vi "Get Logbook Entry.vi"(0 "VISA Session In":refnum<visa-resource-name>="OXYMAT", 1 "Target Address":u8=16 format="%.0x", 2 "Source Address":u8=208 format="%.0x", 7 "Entry":u8, 11 "error in (no error)":errorcluster) -> (4 "VISA Session Out":refnum<visa-resource-name>, 6 "Message Header":T2 {"Source Address" format="%.0x"; "Target Address" format="%.0x"}, 8 "Log Entry":T1 {"Timestamp" format="%<%X %x>T"}, 13 "Success":bool, 15 "error out":errorcluster)   [LabVIEW 2019, in "Siemens ELAN.lvlib"]
doc: "Using the Siemens ELAN protocol, gets the specifed log entry from the addressed analyzer. Also returns a boolean indicating that the addressed device provided a valid response.\n\n$Revision:: 0 $\n$Modtime:: yy-mm-dd hh:mm $\n$Author:: Dboyd $"
uses:
  Siemens ELAN.lvlib
  Message Header.ctl
  Channel Status.ctl
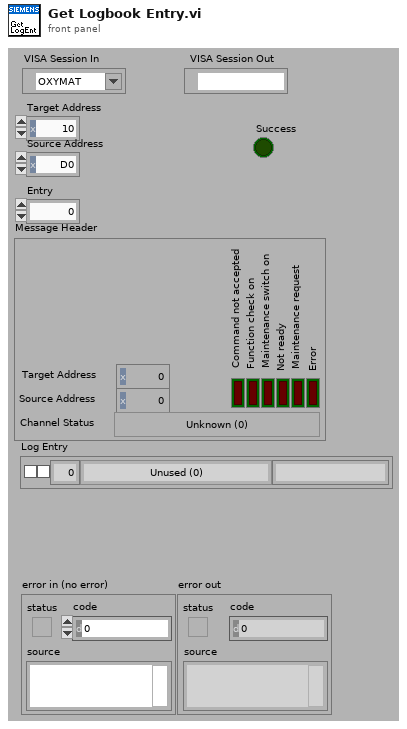
[diagram p1: front panel]
types:
  T1 = cluster{"Entry":u8, "Fault/Maint":enum8{"Unused (0)", "S1 Param Memory", "S2 Chopper/Magnetic Field", "S3 Microflow Sensor", "S4 External Fault", "S5 AnalyzerTemperature", "S6 Field Device Heater", "S7 Measuring Head Temperature", "S8 Pressure Sensor", "S9 Signal Too Large", "Unused (S10)", "S11 Reference Gas Supply", "S12 Mains Power", "Unused (S13)", "S14 Measured Value > Full Scale", "S15 Calibration Aborted", "S16 Sample Flow Too Low", "W1 Calibration Tolerance Violated", "W2 Zero Adjustment Too High", "W3 Slope/Sensitivity Too Small", "W4 Set Clock", "W5 Microflow Sensor", "W6 LCD Temperature", "W7 Analyzer/Receiver Temperature", "W8 Measuring Head Temperature", "W9 External Maintenance Request", "Unknown (W10)", "Unknown (W11)", "W12 Maintenance Check", "Unknown (>28)"}, "Appeared?":bool, "Acknowledged?":bool, "Timestamp":timestamp}
  T2 = typedef "Siemens ELAN.lvlib/Message Header.ctl" = cluster{"Target Address":u8, "Source Address":u8, "Error":bool, "Maintenance request":bool, "Not ready":bool, "Maintenance switch on":bool, "Function check on":bool, "Command not accepted":bool, "Channel Status":T3}
  T3 = typedef "Siemens ELAN.lvlib/Channel Status.ctl" = enum8{"Unknown (0)", "Warm-up", "Pause", "Standby", "Measure", "Zero calibration", "Adjust component slope", "Unknown (7)", "Adjust curve dip", "Adjust linearization sensitivity", "Adjust temperature compensation", "Adjust pressure compensation", "Adjust linearization zero", "Adjust flow sensor", "Autocal", "Adjust phase", "Zero calibration of O2 sensor", "Synchronous zero calibration", "Purging for synchronous zero calibration", "Adjust analog output", "Adjust analog input", "Cleaning", "Unknown (>21)"}
  T4 = enum8{"Unused (0)", "S1 Param Memory", "S2 Chopper/Magnetic Field", "S3 Microflow Sensor", "S4 External Fault", "S5 AnalyzerTemperature", "S6 Field Device Heater", "S7 Measuring Head Temperature", "S8 Pressure Sensor", "S9 Signal Too Large", "Unused (S10)", "S11 Reference Gas Supply", "S12 Mains Power", "Unused (S13)", "S14 Measured Value > Full Scale", "S15 Calibration Aborted", "S16 Sample Flow Too Low", "W1 Calibration Tolerance Violated", "W2 Zero Adjustment Too High", "W3 Slope/Sensitivity Too Small", "W4 Set Clock", "W5 Microflow Sensor", "W6 LCD Temperature", "W7 Analyzer/Receiver Temperature", "W8 Measuring Head Temperature", "W9 External Maintenance Request", "Unknown (W10)", "Unknown (W11)", "W12 Maintenance Check", "Unknown (>28)"}
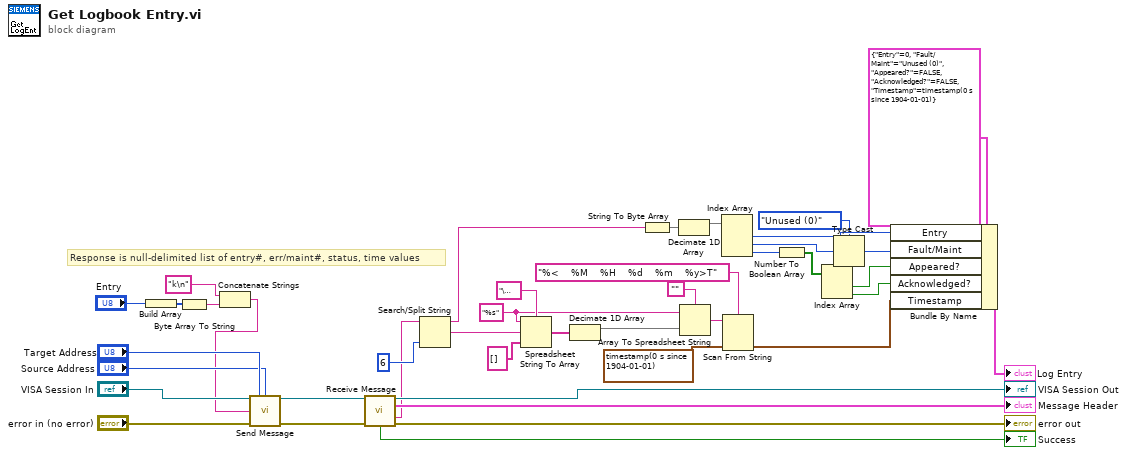
[diagram p0: block diagram]
diagram:
  w22 = "%s" ("format string")
  # "Response is null-delimited list of entry#, err/maint#, status, time values"
  n1 = Build Array("Entry") -> (w11:u8[])
  n2 = Byte Array To String(unsigned byte array=w11) -> (string=w10:string)
  n3 = Concatenate Strings("k\n" ("Command"), w10) -> (w8:string)
  n4 = call "Send Message.vi"("VISA Session In"="VISA Session In", "Target Address"="Target Address", "Source Address"="Source Address", "Command"=w8, "error in (no error)"="error in (no error)") -> ("VISA Session Out"=w41:refnum<visa-resource-name>, "error out"=w40:errorcluster)  [unwired: 8 in, 1 out]
  n5 = call "Receive Message.vi"("VISA Session In"=w41, "error in (no error)"=w40) -> ("VISA Session Out"=→"VISA Session Out":refnum<visa-resource-name>, "Message Header"=→"Message Header":T2, "Response"=w4:string, "Success"=→"Success":bool, "error out"=→"error out":errorcluster)  [unwired: 8 in, 1 out]
  n6 = Search/Split String(string=w4, offset (0)=6) -> (substring before match=w3:string, match + rest of string=w2:string)  [unwired: 1 in, 1 out]
  n7 = Spreadsheet String To Array(delimiter (Tab)="\u0000", format string=w22, spreadsheet string=w2, array type (2D Dbl)=string[] []) -> (array=w23:string[])
  n8 = Decimate 1D Array(w23) -> (w26:string[])  [unwired: 1 out]
  n9 = String To Byte Array(string=w3) -> (unsigned byte array=w7:u8[])
  n10 = Decimate 1D Array(w7) -> (w6:u8[])  [unwired: 1 out]
  n11 = Array To Spreadsheet String(delimiter (Tab)="", array=w26, 3:w22) -> (spreadsheet string=w28:string)
  n12 = Index Array(array=w6) -> (element #1=w20:u8, element #2=w24:u8, element #3=w18:u8)  [unwired: 3 in]
  n13 = Scan From String(format string="%<    %M    %H    %d    %m    %y>T", input string=w28, default 1=timestamp(0 s since 1904-01-01) ("Timestamp")) -> (output 1=w14:timestamp)  [unwired: 2 in, 3 out]
  n14 = Number To Boolean Array(number=w18) -> (Boolean array=w17:bool[])
  n15 = Index Array(array=w17) -> (element #1=w16:bool, element #2=w15:bool)  [unwired: 2 in]
  n16 = Type Cast(type=T4."Unused (0)" ("Fault/Maint"), x=w24) -> (*(type *) &x=w19:T4)
  n17 = Bundle By Name(cluster=T1 {"Entry"=0, "Fault/Maint"=enum."Unused (0)", "Appeared?"=FALSE, "Acknowledged?"=FALSE, "Timestamp"=timestamp(0 s since 1904-01-01)}, "Entry"=w20, "Fault/Maint"=w19, "Appeared?"=w16, "Acknowledged?"=w15, "Timestamp"=w14) -> (→"Log Entry":T1)
